vi "Write Slow FPGA Telem to FIFO.vi"   [LabVIEW 2014]
uses:
  FPGA Telem for Slow Logging.ctl
  FPGA Loads and Shutdown.ctl
  Dash LED Status.ctl
  <vilib>/FPGAPlugInAG/Dynamic/niLvFpga_Close_Dynamic.vi
  <vilib>/rvi/errors/niLvFpgaAdjustHostInterfaceError.vi
  <vilib>/Utility/error.llb/Error Cluster From Error Code.vi
  Global Data.vi
  <vilib>/rvi/interface/common/dynamic/niFpgaDynamicAddResources.vi
  <vilib>/FPGAPlugInAG/sbRIO-9626/niLvFpga_Open_sbRIO-9626.vi
  <vilib>/rvi/interface/nirviCloseFPGA/nirviCloseFPGA.xnode
  <vilib>/rvi/interface/nirviReadWriteControl/nirviReadWriteControl.xnode
  <vilib>/rvi/interface/nirviOpenFPGA/nirviOpenFPGA.xnode
  FPGA Bitfiles/FormulaElectric2_FPGATarget_FPGA_8a5J0mMac2U.lvbitx
  FPGA/Sensor Library/FPGA.vi
  NiFpgaLv.dll
  <vilib>/rvi/interface/Simulation/niFpgaSimulationCallBeginRW.vi
  <vilib>/NI_Real-Time Target Support.lvlib
types:
  T1 = cluster{"read mode":enum16{"polling", "blocking"}, "write mode":enum16{"polling", "blocking"}}
  T2 = typedef "FPGA Telem for Slow Logging.ctl" = cluster{"Chassis Temperature":fxp<+/-,16,9>, "Supply Voltage (V)":fxp<+/-,25,6>, "Motor Controller Dash Switch":bool, "FPGA LED":bool, "Loads & Shutdown":T3, "CPU Load":cluster{"Total (%)":dbl, "Time Critical (%)":dbl, "Timed Structures (%)":dbl, "High (%)":dbl, "Above Normal (%)":dbl, "Normal (%)":dbl, "Background (%)":dbl, "Idle (%)":dbl, "ISR (%)":dbl}, "Time Stamp":timestamp}
  T3 = typedef "FPGA Loads and Shutdown.ctl" = cluster{"RTDS Enable":bool, "TSMS In Status":bool, "Positive AIR Enable":bool, "cRIO Shutdown 2":bool, "cRIO Shutdown 1":bool, "TSMS Out Status":bool, "Coolant Pump":bool, "BMS OK":bool, "IMD In":bool, "BSPD In":bool, "Brake Light Out":bool, "Green LED":T4, "Yellow LED":T4, "Red LED":T4}
  T4 = typedef "Dash LED Status.ctl" = enum16{"Off", "Flashing", "On"}
  T5 = typedef "NI_Real-Time Target Support.lvlib/RT CPU Load.ctl" = cluster{"Total (%)":dbl, "Time Critical (%)":dbl, "Timed Structures (%)":dbl, "High (%)":dbl, "Above Normal (%)":dbl, "Normal (%)":dbl, "Background (%)":dbl, "Idle (%)":dbl, "ISR (%)":dbl}
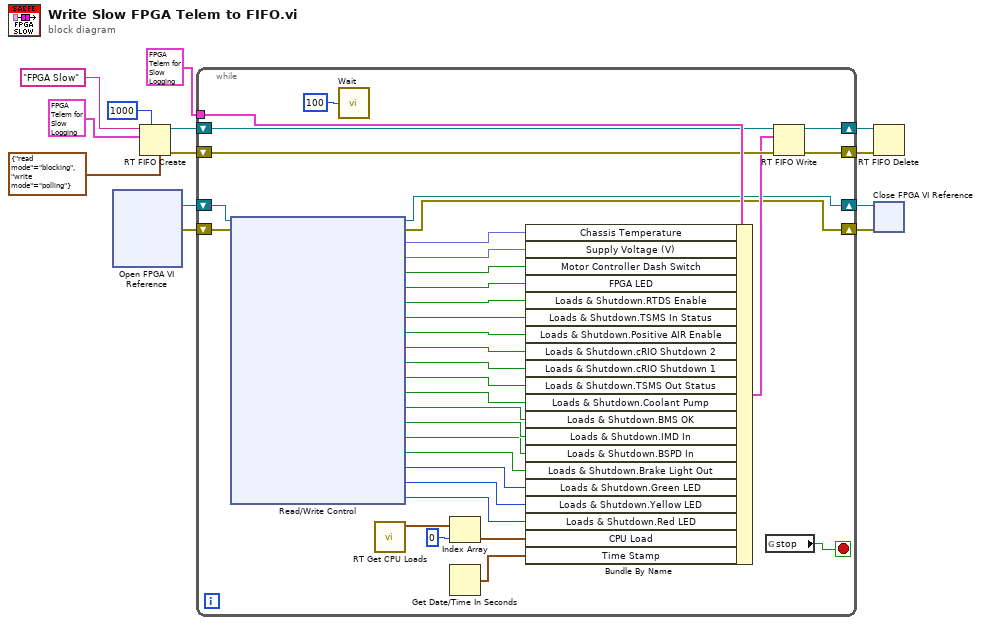
[diagram p0: block diagram]
diagram:
  n1 = xnode "Open FPGA VI Reference"() -> ("FPGA VI Reference Out"=w12:refnum<k20>, "error out"=w11:errorcluster)  [unwired: 2 in]
  n2 = RT FIFO Create(0:"FPGA Slow" ("name (unnamed)"), 1:T2 {"Chassis Temperature"=0.0, "Supply Voltage (V)"=0.0, "Motor Controller Dash Switch"=FALSE, "FPGA LED"=FALSE, "Loads & Shutdown"={"RTDS Enable"=FALSE, "TSMS In Status"=FALSE, "Positive AIR Enable"=FALSE, "cRIO Shutdown 2"=TRUE, "cRIO Shutdown 1"=TRUE, "TSMS Out Status"=FALSE, "Coolant Pump"=FALSE, "BMS OK"=FALSE, "IMD In"=FALSE, "BSPD In"=FALSE, "Brake Light Out"=FALSE, "Green LED"=enum."Off", "Yellow LED"=enum."Off", "Red LED"=enum."Off"}, "CPU Load"={"Total (%)"=0.0, "Time Critical (%)"=0.0, "Timed Structures (%)"=0.0, "High (%)"=0.0, "Above Normal (%)"=0.0, "Normal (%)"=0.0, "Background (%)"=0.0, "Idle (%)"=0.0, "ISR (%)"=0.0}, "Time Stamp"=timestamp(0 s since 1904-01-01)} ("FPGA Logging Telem"), 4:u32 1000 ("size (10)"), 7:T1 {"read mode"=enum."blocking", "write mode"=enum."polling"} ("r/w modes (polling,polling)")) -> (8:w6:refnum<k33>, 11:w5:errorcluster)  [unwired: 4 in, 1 out]
  n3 = while {
    tunnel: T2 {"Chassis Temperature"=0.0, "Supply Voltage (V)"=0.0, "Motor Controller Dash Switch"=FALSE, "FPGA LED"=FALSE, "Loads & Shutdown"={"RTDS Enable"=FALSE, "TSMS In Status"=FALSE, "Positive AIR Enable"=FALSE, "cRIO Shutdown 2"=TRUE, "cRIO Shutdown 1"=TRUE, "TSMS Out Status"=FALSE, "Coolant Pump"=FALSE, "BMS OK"=FALSE, "IMD In"=FALSE, "BSPD In"=FALSE, "Brake Light Out"=FALSE, "Green LED"=enum."Off", "Yellow LED"=enum."Off", "Red LED"=enum."Off"}, "CPU Load"={"Total (%)"=0.0, "Time Critical (%)"=0.0, "Timed Structures (%)"=0.0, "High (%)"=0.0, "Above Normal (%)"=0.0, "Normal (%)"=0.0, "Background (%)"=0.0, "Idle (%)"=0.0, "ISR (%)"=0.0}, "Time Stamp"=timestamp(0 s since 1904-01-01)} ("FPGA Logging Telem") -> [w47]
    shift-right: [w19] -> w3
    shift-left: w6 -> [w22]
    shift-right: [w18] -> w4
    shift-left: w5 -> [w21]
    shift-right: [w16] -> w2
    shift-left: w12 -> [w45]
    shift-right: [w15] -> w1
    shift-left: w11 -> [w44]
    stop <- w46 stop-if-true
    n4 = xnode "Read/Write Control"("FPGA VI Reference In"=w45, "error in"=w44) -> ("FPGA VI Reference Out"=w16:refnum<k20>, "error out"=w15:errorcluster, "Chassis Temperature (C)"=w43:fxp<+/-,33,17>, "Supply Voltage (V)"=w42:fxp<+/-,25,6>, "Motor Controller Dash Switch"=w41:bool, "FPGA LED"=w40:bool, "RTDS Enable"=w39:bool, "TSMS In Status"=w38:bool, "Positive AIR Enable"=w37:bool, "cRIO Shutdown 2"=w36:bool, "cRIO Shutdown 1"=w35:bool, "TSMS Out Status"=w34:bool, "Coolant Pump"=w33:bool, "BMS OK"=w32:bool, "IMD In"=w31:bool, "BSPD In"=w30:bool, "Brake Light Out"=w29:bool, "Green LED"=w28:enum16{"Off", "Flashing", "On"}, "Yellow LED"=w27:enum16{"Off", "Flashing", "On"}, "Red LED"=w26:enum16{"Off", "Flashing", "On"})
    n5 = call "Wait"("Count(mSec)"=u32 100) -> ()  [unwired: 1 out]
    n6 = call <vilib>:"RT Get CPU Loads.vi"() -> ("CPU loads"=w25:T5[])  [unwired: 10 in, 1 out]
    n7 = Index Array(array=w25, index=0) -> (element=w23:T5)
    n8 = Get Date/Time In Seconds() -> (seconds since 1Jan1904=w14:timestamp)
    n9 = Bundle By Name(cluster=w47, "Chassis Temperature"=w43, "Supply Voltage (V)"=w42, "Motor Controller Dash Switch"=w41, "FPGA LED"=w40, "Loads & Shutdown.RTDS Enable"=w39, "Loads & Shutdown.TSMS In Status"=w38, "Loads & Shutdown.Positive AIR Enable"=w37, "Loads & Shutdown.cRIO Shutdown 2"=w36, "Loads & Shutdown.cRIO Shutdown 1"=w35, "Loads & Shutdown.TSMS Out Status"=w34, "Loads & Shutdown.Coolant Pump"=w33, "Loads & Shutdown.BMS OK"=w32, "Loads & Shutdown.IMD In"=w31, "Loads & Shutdown.BSPD In"=w30, "Loads & Shutdown.Brake Light Out"=w29, "Loads & Shutdown.Green LED"=w28, "Loads & Shutdown.Yellow LED"=w27, "Loads & Shutdown.Red LED"=w26, "CPU Load"=w23, "Time Stamp"=w14) -> (w20:T2)
    n10 = global read "Global Data.vi" "stop"() -> (w46:bool)
    n11 = RT FIFO Write(0:w22, 1:w20, 3:w21) -> (8:w19:refnum<k33>, 11:w18:errorcluster)  [unwired: 2 in, 2 out]
  }
  n12 = RT FIFO Delete(0:w3, 3:w4) -> ()  [unwired: 1 in, 1 out]
  n13 = xnode "Close FPGA VI Reference"("FPGA VI Reference In"=w2, "error in"=w1) -> ()  [unwired: 1 out]
